vi "AuMT8852B Fixed Path Offset.vi"(5 "Offset (0)":dbl format="%.1f", 7 "Set/Get (Set)":enum16{"Set", "Get"}(ring), 8 "error in (no error)":errorcluster, 10 "Script (3)":i32=3, 11 "VISA session":refnum<visa-resource-name>) -> (0 "error out":errorcluster, 2 "error code":i32, 3 "VISA session out":refnum<visa-resource-name>, 4 "Offset out":dbl format="%.1f")   [LabVIEW 2017]
doc: "Anritsu MT8852B Bluetooth Tester\n\nSends or receives the fixed offset that will be applied to the transmitter power. For use when the Path Offset Mode is set to Fixed.\n\nINPUTS\nSet/Get - whether the value is being sent to or retrieved from the instrument.\nScript - the script number to configure.\nOffset - fixed path offset to use.\n\nOUTPUTS\nOffset out - fixed path offset currently being used."
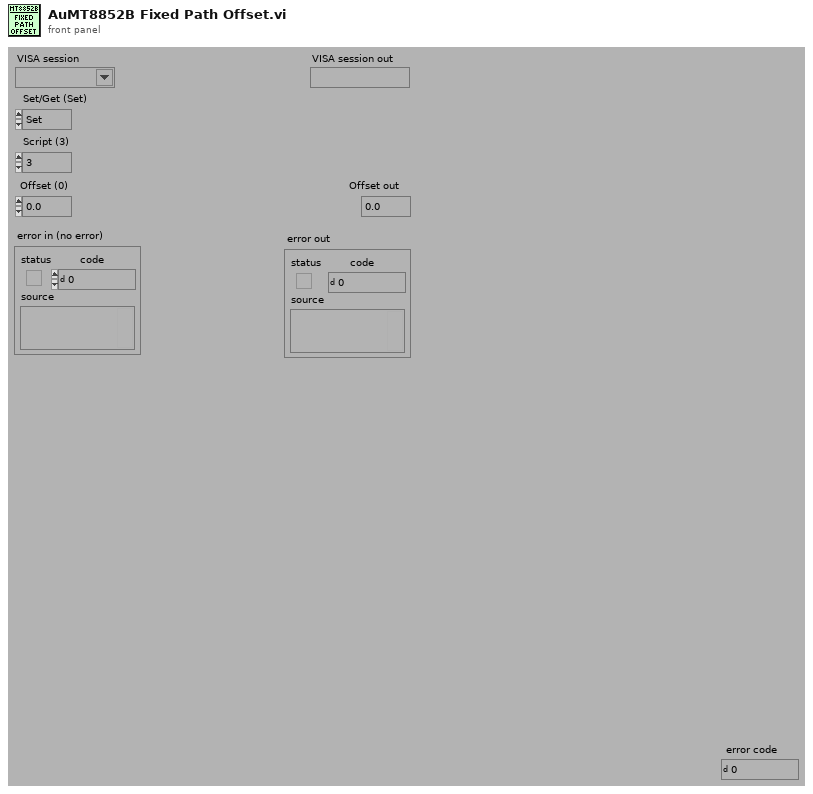
[diagram p1: front panel]
types:
  T1 = enum16{"Simulate", "Range check", "Cache", "Query instrument status"}
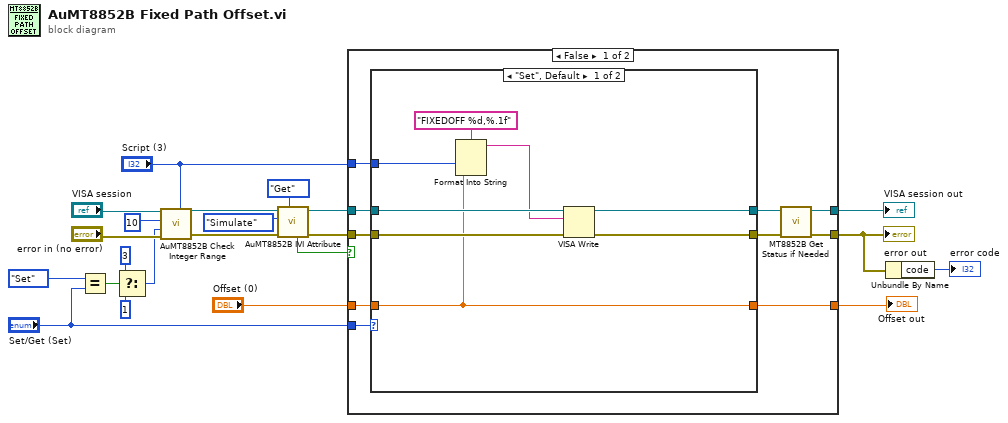
[diagram p0: block diagram]
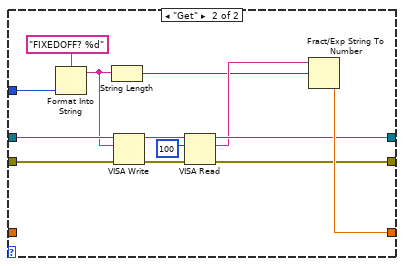
[diagram p2: hidden frame]
diagram:
  n1 = Equal?(x=enum16{"Set", "Get"}."Set", y="Set/Get (Set)") -> (x = y?=w6:bool)
  n2 = Select(t=3, s=w6, f=1) -> (s? t:f=w3:i32)
  n3 = call <instrlib>:"AuMT8852B Check Integer Range.vi"("Value (0)"="Script (3)", "error in (no error)"="error in (no error)", "Lower limit (-1)"=w3, "Upper limit (1)"=10, "VISA session"="VISA session") -> ("error out"=w15:errorcluster, "VISA session out"=w14:refnum<visa-resource-name>)  [unwired: 5 in]
  n4 = call <instrlib>:"AuMT8852B IVI Attribute.vi"("Set/Get (Set)"=enum16{"Set", "Get"}."Get", "error in (no error)"=w15, "Flag (Simulate)"=T1."Simulate", "VISA session"=w14) -> ("error out"=w20:errorcluster, "VISA session out"=w21:refnum<visa-resource-name>, "Value out"=w17:bool)  [unwired: 5 in]
  n5 = case shown="False" w17 {
    tunnel: [w23 w56] -> w22
    tunnel: [w24 w55] -> w1
    tunnel: w21 -> [w32 w56]
    tunnel: w20 -> [w31 w55]
    tunnel: [w30 w54] -> w16
    tunnel: "Script (3)" -> [w29 _]
    tunnel: "Set/Get (Set)" -> [w28 _]
    tunnel: "Offset (0)" -> [w27 w54]
    frame False {
      n6 = case shown="\"Set\", Default" w28 {
        tunnel: w32 -> [w38 w53]
        tunnel: w31 -> [w39 w52]
        tunnel: [w33 w43] -> w26
        tunnel: [w36 w45] -> w30
        tunnel: w29 -> [w37 w49]
        tunnel: w27 -> [w36 _]
        tunnel: [w34 w44] -> w25
        frame "Set", Default {
          n7 = Format Into String(format string="FIXEDOFF %d,%.1f" ("Command ()"), w37, w36) -> (resulting string=w35:string)  [unwired: 2 in, 1 out]
          n8 = VISA Write(VISA resource name=w38, write buffer=w35, error in (no error)=w39) -> (VISA resource name out=w34:refnum<visa-resource-name>, error out=w33:errorcluster)  [unwired: 1 out]
        }
        frame "Get" {
          n9 = Format Into String(format string="FIXEDOFF? %d" ("Format String"), w49) -> (resulting string=w46:string)  [unwired: 2 in, 1 out]
          n10 = String Length(string=w46) -> (length=w41:i32)
          n11 = VISA Write(VISA resource name=w53, write buffer=w46, error in (no error)=w52) -> (VISA resource name out=w50:refnum<visa-resource-name>, error out=w51:errorcluster)  [unwired: 1 out]
          n12 = VISA Read(VISA resource name=w50, byte count=u32 100 ("byte count (0)"), error in (no error)=w51) -> (VISA resource name out=w44:refnum<visa-resource-name>, read buffer=w42:string, error out=w43:errorcluster)  [unwired: 1 out]
          n13 = Fract/Exp String To Number(string=w42, offset=w41) -> (number=w45:dbl)  [unwired: 2 in, 1 out]
        }
      }
      n14 = call <instrlib>:"MT8852B Get Status if Needed.vi"("error in (no error)"=w26, "VISA session"=w25) -> ("error out"=w24:errorcluster, "VISA session out"=w23:refnum<visa-resource-name>)  [unwired: 8 in]
    }
    frame True {
      (unwired) "" ("Response")
    }
  }
  "error out" <- w1
  "VISA session out" <- w22
  "Offset out" <- w16
  n15 = Unbundle By Name(w1) -> ("code"=→"error code":i32)
